vi "CameraAngle.vi"(4 "MinAngle":dbl, 6 "MaxAngle":dbl, 7 "joystickWheel":dbl, 9 "POT VALUE AT 80*":dbl, 10 "POT VALUE AT 50*":dbl, 11 "Pot Value":dbl) -> (3 "ServoAngle":dbl)   [LabVIEW 2011]
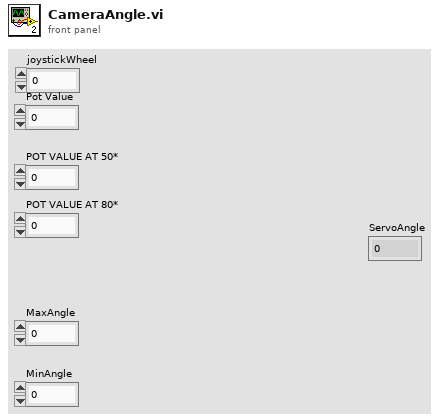
[diagram p1: front panel]
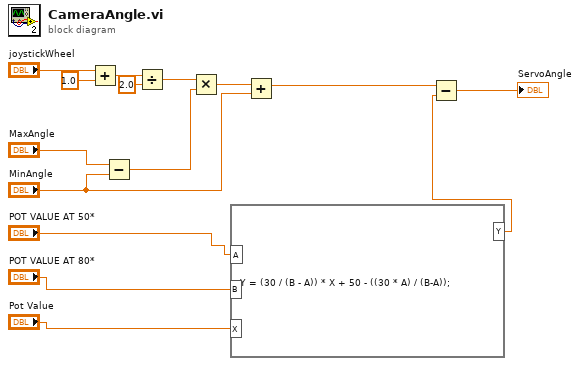
[diagram p0: block diagram]
diagram:
  n1 = Add(x="joystickWheel", y=1.0) -> (x+y=w14:dbl)
  n2 = Subtract(x="MaxAngle", y="MinAngle") -> (x-y=w10:dbl)
  n3 = Divide(x=w14, y=2.0) -> (x/y=w11:dbl)
  n4 = Multiply(x=w11, y=w10) -> (x*y=w9:dbl)
  n5 = formula code="Y = (30 / (B - A)) * X + 50 - ((30 * A) / (B-A));"("X"="Pot Value", "B"="POT VALUE AT 80*", "A"="POT VALUE AT 50*") -> ("Y"=w2:dbl)
  n6 = Add(x=w9, y="MinAngle") -> (x+y=w3:dbl)
  n7 = Subtract(x=w3, y=w2) -> (x-y=→"ServoAngle":dbl)
